vi "Probe - SysAPI.vi"(8 "error in (no error)":errorcluster) -> (0 "error out":errorcluster, 1 "SysAPI Information":T2[](array[typedef]), 2 "NI Software Packages":T1[](array[typedef]))   [LabVIEW 2021, in "Acquisition.lvlib"]
doc: "Use SysAPI to detect the installed software and discovered IO devices on the running Host system. Return an array of 'Software Package's and an array of 'Host IO Resource's."
uses:
  Acquisition.lvlib
  Host IO Resource.ctl
  Host Software Package.ctl
  <vilib>/nisyscfg/Component Types.ctl
  <vilib>/nisyscfg/Get Installed Components.vi
  <vilib>/nisyscfg/Close (System).vi
  <vilib>/nisyscfg/nisyscfg.lvlib
  <resource>/objmgr/nisysapi.rc
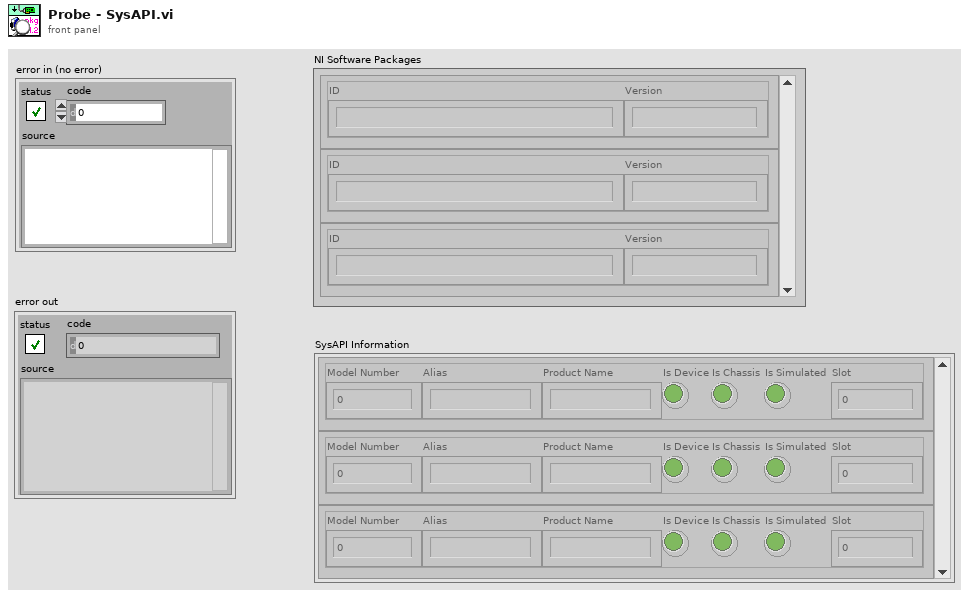
[diagram p1: front panel]
types:
  T1 = typedef "Acquisition.lvlib/Host Software Package.ctl" = cluster{"ID":string, "Version":string}
  T2 = typedef "Acquisition.lvlib/Host IO Resource.ctl" = cluster{"Model Number":u32, "Alias":string, "Product Name":string, "Is Device":bool, "Is Chassis":bool, "Is Simulated":bool, "Slot":i32}
  T3 = typedef "nisyscfg.lvlib/Component Types.ctl" = u32
  T4 = typedef "nisyscfg.lvlib/Software 1.2.ctl" = cluster{"title":string, "description":string, "ID":string, "version":string, "component type":T5}
  T5 = typedef "nisyscfg.lvlib/Component Type.ctl" = u32
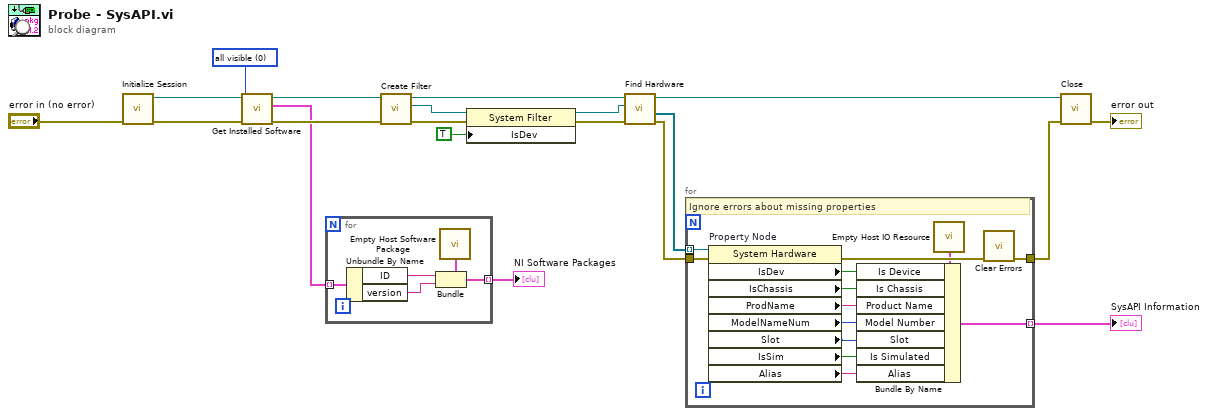
[diagram p0: block diagram]
diagram:
  w16 = T3 0 items=["all visible", "all including hidden", "standard only", "startup only"] ("Item Types (all visible)")
  n1 = call <vilib>:"Initialize Session.vi"("error in (no error)"="error in (no error)") -> ("error out"=w7:errorcluster, "Session out"=w17:refnum<k21>)  [unwired: 9 in]
  n2 = call-poly <vilib>:"Get Installed Software.vi"("error in (no error)"=w7, "Item Types (all visible)"=w16, "Session in"=w17) -> ("error out"=w15:errorcluster, "Software Components"=w6:T4[], "Session out"=w14:refnum<k21>)  [unwired: 6 in]
  n3 = for {
    tunnel: w6 -> [w25] mode=indexing
    tunnel: [w23] -> w5 mode=indexing
    n4 = Unbundle By Name(w25) -> ("ID"=w22:string, "version"=w24:string)
    n5 = call "Empty Host Software Package.vi"() -> ("Software Package"=w21:T1)
    n6 = Bundle(cluster=w21, "ID"=w22, "Version"=w24) -> (w23:T1)
  }
  "NI Software Packages" <- w5
  n7 = call <vilib>:"Create Filter.vi"("error in (no error)"=w15, "Session in"=w14) -> ("error out"=w11:errorcluster, "Filter out"=w13:refnum<k20>, "Session out"=w12:refnum<k21>)  [unwired: 7 in]
  n8 = property on="Property Node" class="System Filter"(reference=w13, error in=w11, "IsDev"=TRUE ("Is Device")) -> (reference out=w9:refnum<k20>, error out=w10:errorcluster)
  n9 = call <vilib>:"Find Hardware.vi"("error in (no error)"=w10, "Filter in"=w9, "Session in"=w12) -> ("error out"=w3:errorcluster, "Resources out"=w18:refnum<k20>[], "Session out"=w19:refnum<k21>)  [unwired: 5 in, 1 out]
  n10 = for {
    tunnel: w18 -> [w38] mode=indexing
    tunnel: w3 -> [w37]
    tunnel: [w35] -> w2
    tunnel: [w26] -> w1 mode=indexing
    # "Ignore errors about missing properties"
    n11 = property on="Property Node" class="System Hardware"(reference=w38, error in=w37) -> (error out=w36:errorcluster, "IsDev"=w27:bool, "IsChassis"=w28:bool, "ProdName"=w29:string, "ModelNameNum"=w30:u32, "Slot"=w31:i32, "IsSim"=w32:bool, "Alias"=w33:string)  [unwired: 1 out]
    n12 = call "Empty Host IO Resource.vi"() -> ("Host IO Resource"=w34:T2)
    n13 = Bundle By Name(cluster=w34, "Is Device"=w27, "Is Chassis"=w28, "Product Name"=w29, "Model Number"=w30, "Slot"=w31, "Is Simulated"=w32, "Alias"=w33) -> (w26:T2)
    n14 = call <vilib>:"Clear Errors.vi"("error in (no error)"=w36) -> ("error out"=w35:errorcluster)  [unwired: 5 in, 1 out]
  }
  "SysAPI Information" <- w1
  n15 = call-poly <vilib>:"Close.vi"("error in (no error)"=w2, "Session in"=w19) -> ("error out"=→"error out":errorcluster)  [unwired: 9 in]
